vi "One 32-bit Port Digital Output.vi"(2 "Packet":u64, 4 "32-Bit DO Port":refnum<k21>="Chassis2/Mod4/DIO31:0") -> ()   [LabVIEW 2009]
uses:
  <vilib>/eio/EIONode/EIONode.xnode
  <vilib>/rvi/eio/nirviEIOImplementation/nirviEIOImplementation.xnode
  <vilib>/rvi/eio/common/nirviEmuTemplateMethod_noerrors.vi
  <vilib>/rvi/eio/common/nirviEmuClasses.ctl
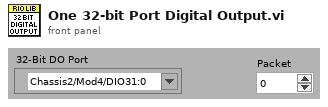
[diagram p1: front panel]
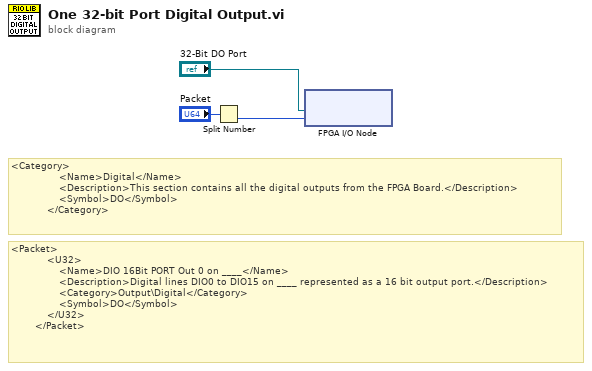
[diagram p0: block diagram]
diagram:
  # "<Packet>\n            <U32>\n                <Name>DIO 16Bit PORT Out 0 on ____</Name>\n                <Description>Digital lines DIO0 to DIO15 on ____ represented as a 16 bit output port.</Description>\n                <Category>Output\\Digital</Category>\n                <Symbol>DO</Symbol>\n            </U32>\n        </Packet>"
  # "<Category>\n                <Name>Digital</Name>\n                <Description>This section contains all the digital outputs from the FPGA Board.</Description>\n                <Symbol>DO</Symbol>\n            </Category>"
  n1 = Split Number(x="Packet") -> (lo(x)=w1:u32)  [unwired: 1 out]
  n2 = xnode "FPGA I/O Node"("I/O Item"=w1, "FPGA I/O In"="32-Bit DO Port") -> ()  [unwired: 1 out]
